vi "LVString to Unicode String.vi"(8 "错误输入":errorcluster, 11 "Input String":string) -> (0 "错误输出":errorcluster, 3 "Output String":string)   [LabVIEW 2012, in "Encoding.lvlib"]
uses:
  Encoding.lvlib
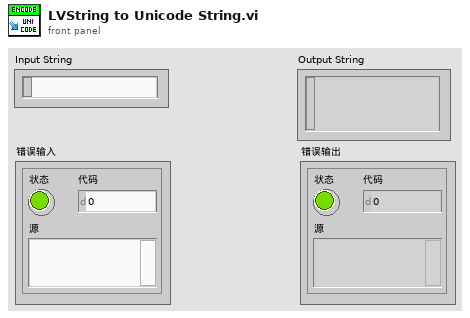
[diagram p1: front panel]
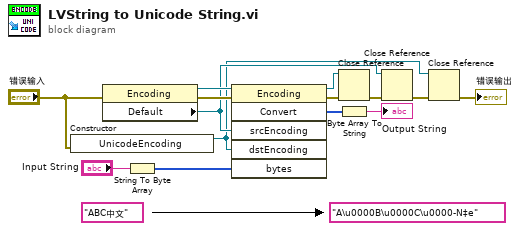
[diagram p0: block diagram]
diagram:
  (unwired) "A\u0000B\u0000C\u0000-N‡e" ("Output String")
  (unwired) "ABC中文" ("Input String")
  n1 = constructor class="UnicodeEncoding"(error in="错误输入") -> (reference out=w5:refnum<k24>)  [unwired: 2 in, 2 out]
  n2 = property class="Encoding"(error in="错误输入") -> (reference out=w10:refnum<k24>, error out=w11:errorcluster, "Default"=w9:refnum<k24>)  [unwired: 1 in]
  n3 = String To Byte Array(string="Input String") -> (unsigned byte array=w13:u8[])
  n4 = invoke class="Encoding" method="Convert"(reference=w10, error in=w11, "srcEncoding"=w9, "dstEncoding"=w5, "bytes"=w13) -> (reference out=w2:refnum<k24>, error out=w1:errorcluster, "Convert"=w3:u8[])  [unwired: 1 in, 3 out]
  n5 = Close Reference(reference=w2, error in (no error)=w1) -> (error out=w8:errorcluster)
  n6 = Byte Array To String(unsigned byte array=w3) -> (string=→"Output String":string)
  n7 = Close Reference(reference=w9, error in (no error)=w8) -> (error out=w7:errorcluster)
  n8 = Close Reference(reference=w5, error in (no error)=w7) -> (error out=→"错误输出":errorcluster)
